vi "Switch Control.vi"(0 "VISA resource name":refnum<visa-resource-name>, 1 "Pin":u8 max=7 step=1, 2 "Enable Input Terminal (F: Off)":bool, 3 "error in (no error)":errorcluster) -> (7 "VISA resource name out":refnum<visa-resource-name>, 10 "error out":errorcluster)   [LabVIEW 2022 SP3, in "usbtmc_scpi_labtool.lvlib"]
doc: "Enables or Disables the output of power supply.\n\n* Output Enable (T:Enable) : \n If true it Switches ON the power supply Output else doesn't respond."
uses:
  usbtmc_scpi_labtool.lvlib
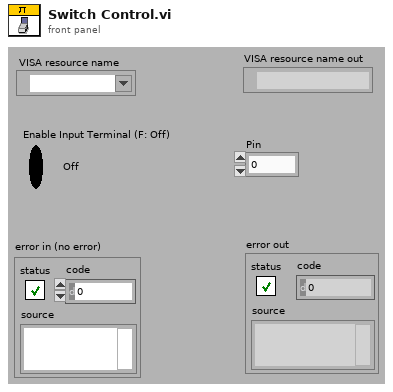
[diagram p1: front panel]
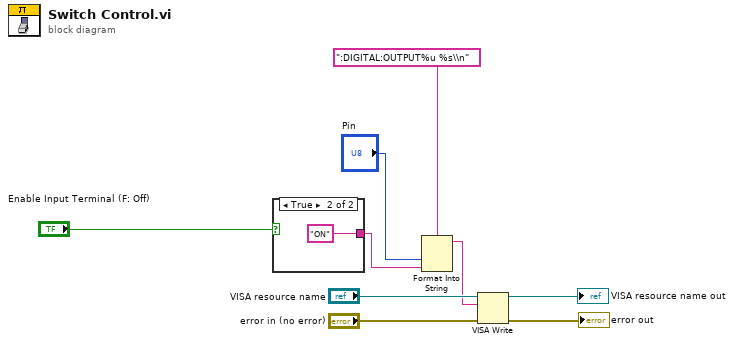
[diagram p0: block diagram]
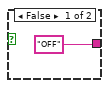
[diagram p2: hidden frame]
diagram:
  n1 = case shown="True" "Enable Input Terminal (F: Off)" {
    tunnel: ["OFF" "ON"] -> w2
    frame False {
    }
    frame True {
    }
  }
  n2 = Format Into String(format string=":DIGITAL:OUTPUT%u %s\\n", "Pin", w2) -> (resulting string=w6:string)  [unwired: 2 in, 1 out]
  n3 = VISA Write(VISA resource name="VISA resource name", write buffer=w6, error in (no error)="error in (no error)") -> (VISA resource name out=→"VISA resource name out":refnum<visa-resource-name>, error out=→"error out":errorcluster)  [unwired: 1 out]
